vi "Swerve Wheel 6181.vi"(2 "Wheel":T2(ring), 4 "Inputs":dbl[](array[numeric])) -> (0 "Speed":dbl)   [LabVIEW 2020]
doc: "This vi is used to calculate and control the position of the swerve wheels and the commanded output to the drive motors."
uses:
  <vilib>/Rock Robotics/WPI/ThirdParty/Phoenix-LabVIEW/CANCoder/Get/CTRE_Phoenix_CANcoder_GetSensorData.vi
  <vilib>/addons/control/pid/pid.llb/PID (DBL).vi
  <vilib>/addons/control/pid/NI_PID_pid.lvlib
panel:
  in  "PID gains":T1={"proportional gain (Kc)"=0.012, "integral time (Ti, min)"=0.0, "derivative time (Td, min)"=0.0}
  in  "BR":dbl=269.0 format="%#_13g"
  in  "BL":dbl=77.0 format="%#_13g"
  in  "FR":dbl=264.0 format="%#_13g"
  in  "FL":dbl=184.0 format="%#_13g"
  # "Steering Motor Encoder Offsets"
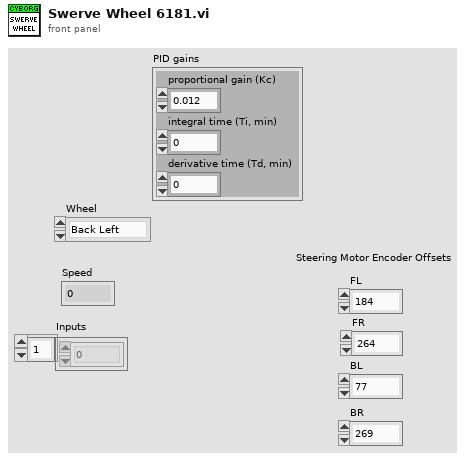
[diagram p1: front panel]
types:
  T1 = cluster{"proportional gain (Kc)":dbl, "integral time (Ti, min)":dbl, "derivative time (Td, min)":dbl}
  T2 = enum16{"Back Left", "Back Right", "Front Left", "Front Right"}
  T3 = enum16{"Z", "Y", "X", "Width/2", "Length/2", "Max"}
  T4 = typedef "CTRE_Phoenix_CANcoder_DeviceRef.ctl" = cluster{"DeviceStatus":errorcluster, "Device Number":u8, "Handle":u64, "UsageFrame":u32, "Library Path":path}
  T5 = typedef "WPI_MotorControlDeviceRef.ctl" = cluster{"DeviceStatus":errorcluster, "Type":T6, "PWM":cluster{"PWM Channel":T7, "DeadBand":T8}, "CAN":cluster{"Device Number":u8, "SetOutput VI Ref":variant, "GetOutput VI Ref":variant, "Enable VI Ref":variant, "Disable VI Ref":variant, "Data":variant}, "Invert":bool, "DIO PWM":cluster{"PWM \"Enable\" Channel":T7, "DIOChannel":T9, "PWM Rate":dbl}}
  T6 = typedef "WPI_MotorControlType.ctl" = enum16{"PWM", "CAN", "DIO PWM"}
  T7 = typedef "FPGA_DIOPWMChannel.ctl" = enum8{"PWM 0", "PWM 1", "PWM 2", "PWM 3", "PWM 4", "PWM 5", "PWM 6", "PWM 7", "PWM 8", "PWM 9", "PWM MXP 0", "PWM MXP 1", "PWM MXP 2", "PWM MXP 3", "PWM MXP 4", "PWM MXP 5", "PWM MXP 6", "PWM MXP 7", "PWM MXP 8", "PWM MXP 9", "Invalid"}
  T8 = typedef "WPI_PWMDeadband.ctl" = cluster{"Name":string, "maxPositivePwm":i32, "minPositivePwm":i32, "centerPwm":i32, "maxNegativePwm":i32, "minNegativePwm":i32, "angularRange":u16}
  T9 = typedef "FPGA_DIOChannel.ctl" = enum8{"DIO 0", "DIO 1", "DIO 2", "DIO 3", "DIO 4", "DIO 5", "DIO 6", "DIO 7", "DIO 8", "DIO 9", "DIO MXP 0", "DIO MXP 1", "DIO MXP 2", "DIO MXP 3", "DIO MXP 4", "DIO MXP 5", "DIO MXP 6", "DIO MXP 7", "DIO MXP 8", "DIO MXP 9", "DIO MXP 10", "DIO MXP 11", "DIO MXP 12", "DIO MXP 13", "DIO MXP 14", "DIO MXP 15", "SPI Port CS1", "SPI Port CS2", "SPI Port CS3", "SPI Port MISO", "SPI Port MOSI", "Invalid"}
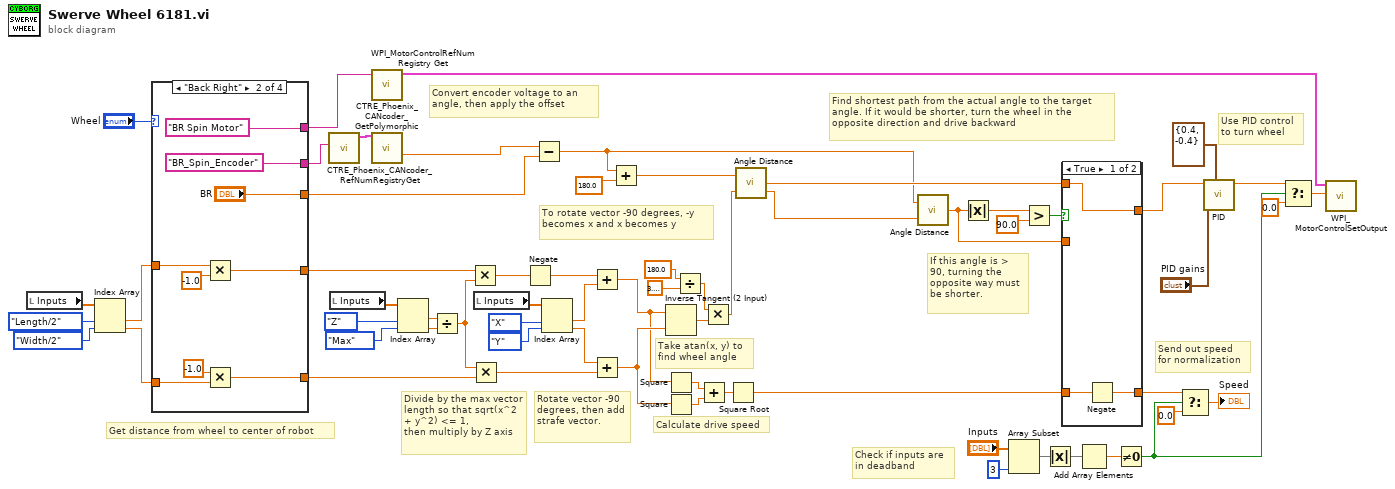
[diagram p0: block diagram]
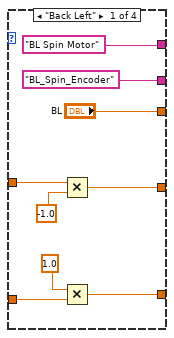
[diagram p3: hidden frame]
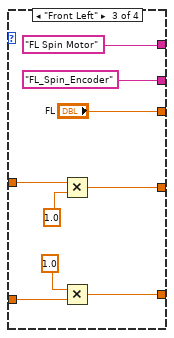
[diagram p4: hidden frame]
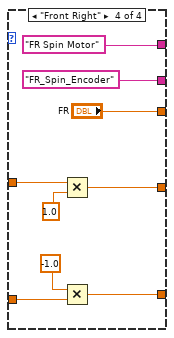
[diagram p5: hidden frame]
diagram:
  # "To rotate vector -90 degrees, -y becomes x and x becomes y"
  # "Divide by the max vector length so that sqrt(x^2 + y^2) <= 1,\nthen multiply by Z axis"
  # "Send out speed\nfor normalization"
  # "Check if inputs are\nin deadband"
  # "Convert encoder voltage to an angle, then apply the offset"
  # "If this angle is > 90, turning the opposite way must be shorter."
  # "Use PID control\nto turn wheel"
  # "Find shortest path from the actual angle to the target angle. If it would be shorter, turn the wheel in the opposite direction and drive backward"
  # "Take atan(x, y) to find wheel angle"
  # "Calculate drive speed"
  # "Rotate vector -90 degrees, then add strafe vector."
  # "Get distance from wheel to center of robot"
  n1 = local read "Inputs"() -> (w20:dbl[])
  n2 = Index Array(array=w20, index #1=T3."Length/2", index #2=T3."Width/2") -> (element #1=w19:dbl, element #2=w18:dbl)
  n3 = case shown="\"Back Right\"" "Wheel" {
    tunnel: ["BL_Spin_Encoder" "BR_Spin_Encoder" "FL_Spin_Encoder" "FR_Spin_Encoder"] -> w7
    tunnel: ["BL Spin Motor" "BR Spin Motor" "FL Spin Motor" "FR Spin Motor"] -> w6
    tunnel: ["BL" "BR" "FL" "FR"] -> w45
    tunnel: w19 -> [w68 w77 w86 w95]
    tunnel: w18 -> [w66 w75 w84 w93]
    tunnel: [w65 w74 w83 w92] -> w34
    tunnel: [w64 w73 w82 w91] -> w33
    frame "Back Left" {
      n4 = Multiply(x=w68, y=-1.0) -> (x*y=w65:dbl)
      n5 = Multiply(x=1.0 ("y"), y=w66) -> (x*y=w64:dbl)
    }
    frame "Back Right" {
      n6 = Multiply(x=w77, y=-1.0) -> (x*y=w74:dbl)
      n7 = Multiply(x=-1.0 ("y"), y=w75) -> (x*y=w73:dbl)
    }
    frame "Front Left" {
      n8 = Multiply(x=w86, y=1.0) -> (x*y=w83:dbl)
      n9 = Multiply(x=1.0 ("y"), y=w84) -> (x*y=w82:dbl)
    }
    frame "Front Right" {
      n10 = Multiply(x=w95, y=1.0) -> (x*y=w92:dbl)
      n11 = Multiply(x=-1.0 ("y"), y=w93) -> (x*y=w91:dbl)
    }
  }
  n12 = call <vilib>:"CTRE_Phoenix_CANcoder_RefNumRegistryGet.vi"("refnum name"=w7) -> ("CTRE_CANcoder_DeviceRef"=w46:T4)  [unwired: 9 in, 1 out]
  n13 = local read "Inputs"() -> (w32:dbl[])
  n14 = call <vilib>:"WPI_MotorControlRefNum Registry Get.vi"("refnum name"=w6) -> ("MotorControlDevRef"=w60:T5)  [unwired: 9 in, 1 out]
  n15 = call-poly <vilib>:"CTRE_Phoenix_CANcoder_GetPolymorphic.vi"("CTRE_CANcoder_DeviceRef"=w46) -> ("Absolute Position"=w3:dbl)  [unwired: 10 in, 4 out]
  n16 = Index Array(array=w32, index #1=T3."Z", index #2=T3."Max") -> (element #1=w30:dbl, element #2=w31:dbl)
  n17 = Divide(x=w30, y=w31) -> (x/y=w29:dbl)
  n18 = Multiply(x=w34, y=w29) -> (x*y=w16:dbl)
  n19 = Multiply(x=w29, y=w33) -> (x*y=w26:dbl)
  n20 = local read "Inputs"() -> (w28:dbl[])
  n21 = Negate(x=w16) -> (-x=w15:dbl)
  n22 = Subtract(x=w3, y=w45) -> (x-y=w4:dbl)
  n23 = Index Array(array=w28, index #1=T3."X", index #2=T3."Y") -> (element #1=w24:dbl, element #2=w25:dbl)
  n24 = Add(x=w15, y=w24) -> (x+y=w22:dbl)
  n25 = Add(x=w25, y=w26) -> (x+y=w23:dbl)
  n26 = Add(x=w4, y=180.0 ("f")) -> (x+y=w42:dbl)
  n27 = Inverse Tangent (2 Input)(1:w23, 2:w22) -> (0:w58:dbl)
  n28 = Square(x=w22) -> (x^2=w27:dbl)
  n29 = Square(x=w23) -> (x^2=w57:dbl)
  n30 = Divide(x=180.0 ("y"), y=3.141592653589793) -> (x/y=w55:dbl)
  n31 = Add(x=w27, y=w57) -> (x+y=w56:dbl)
  n32 = Multiply(x=w55, y=w58) -> (x*y=w17:dbl)
  n33 = Square Root(x=w56) -> (sqrt(x)=w49:dbl)
  n34 = call "Angle Distance.vi"("target angle"=w17, "current angle"=w42) -> ("distance"=w8:dbl)
  n35 = call "Angle Distance.vi"("target angle"=w17, "current angle"=w4) -> ("distance"=w50:dbl)
  n36 = Absolute Value(x=w50) -> (abs(x)=w51:dbl)
  n37 = Array Subset(array="Inputs", length=3) -> (w41:dbl[])  [unwired: 1 in]
  n38 = Greater?(x=w51, y=90.0) -> (0:w37:bool)
  n39 = Absolute Value(x=w41) -> (abs(x)=w35:dbl[])
  n40 = case shown="True" w37 {
    tunnel: w8 -> [w99 _]
    tunnel: w50 -> [_ w103]
    tunnel: [w100 w102] -> w40
    tunnel: w49 -> [w101 w102]
    tunnel: [w99 w103] -> w47
    frame True {
      n41 = Negate(x=w101) -> (-x=w100:dbl)
    }
    frame False {
    }
  }
  n42 = Add Array Elements(numeric array=w35) -> (sum=w59:dbl)
  n43 = Not Equal To 0?(x=w59) -> (x != 0?=w36:bool)
  n44 = Select(t=w40, s=w36, f=0.0) -> (s? t:f=→"Speed":dbl)
  n45 = call-poly <vilib>:"PID.vi"("output range"=cluster{"output high":dbl, "output low":dbl} {"output high"=0.4, "output low"=-0.4}, "PID gains"="PID gains", "setpoint"=w47) -> ("output"=w1:dbl)  [unwired: 7 in, 1 out]
  n46 = Select(t=w1, s=w36, f=0.0) -> (s? t:f=w44:dbl)
  n47 = call <vilib>:"WPI_MotorControlSetOutput.vi"("Output"=w44, "MotorControlDevRef"=w60) -> ()  [unwired: 7 in, 3 out]
